vi "Create AO waveforms Parallel.vi"(9 "sampling info":cluster{"Fs":dbl, "#s":dbl}={"Fs"=1000.0, "#s"=1000.0} {"Fs" format="%.2p"}, 10 "reset signal":bool, 11 "Cluster":T1={"AO amp (V)"=[0.001, 2e-08, 0.001, 0.001, 0.001, 2e-08, 0.0, 0.0], "AO DC (V)"=[0.0, 0.0, 0.0, 0.0, 0.0, 0.0, 0.0, 0.0], "AO f (Hz)"=[13.0, 13.0, 13.0, 13.0, 13.0, 13.0, 13.0, 13.0], "AO phi (deg)"=[0.0, 0.0, 0.0, 0.0, 0.0, 0.0, 0.0, 0.0], "REF f (Hz)"=[13.0, 13.0, 13.0, 13.0, 13.0, 13.0, 13.0, 13.0], "function"=[enum."Sine Wave", enum."Sine Wave", enum."Sine Wave", enum."Sine Wave", enum."Sine Wave", enum."Sine Wave", enum."Sine Wave", enum."Sine Wave"], "REF phi (deg)"=[0.0, 0.0, 0.0, 0.0, 0.0, 0.0, 0.0, 0.0]} {"AO DC (V)" format="%#_6p"; "AO amp (V)" format="%#_6p"}) -> (1 "AO Array":waveform(dbl)[](array[waveform]))   [LabVIEW 2013]
uses:
  <vilib>/measure/NI_MABase.lvlib
panel:
  out "Cluster out":T1={"AO amp (V)"=[0.001, 2e-08, 0.001, 0.001, 0.001, 2e-08, 0.0, 0.0], "AO DC (V)"=[0.0, 0.0, 0.0, 0.0, 0.0, 0.0, 0.0, 0.0], "AO f (Hz)"=[13.0, 13.0, 13.0, 13.0, 13.0, 13.0, 13.0, 13.0], "AO phi (deg)"=[0.0, 0.0, 0.0, 0.0, 0.0, 0.0, 0.0, 0.0], "REF f (Hz)"=[13.0, 13.0, 13.0, 13.0, 13.0, 13.0, 13.0, 13.0], "function"=[enum."Sine Wave", enum."Sine Wave", enum."Sine Wave", enum."Sine Wave", enum."Sine Wave", enum."Sine Wave", enum."Sine Wave", enum."Sine Wave"], "REF phi (deg)"=[0.0, 0.0, 0.0, 0.0, 0.0, 0.0, 0.0, 0.0]} {"AO DC (V)" format="%#_6p"; "AO amp (V)" format="%#_6p"}
  out "Waveform Graph":waveform(dbl)[](graph)
  out "phase out":dbl[](array[numeric])
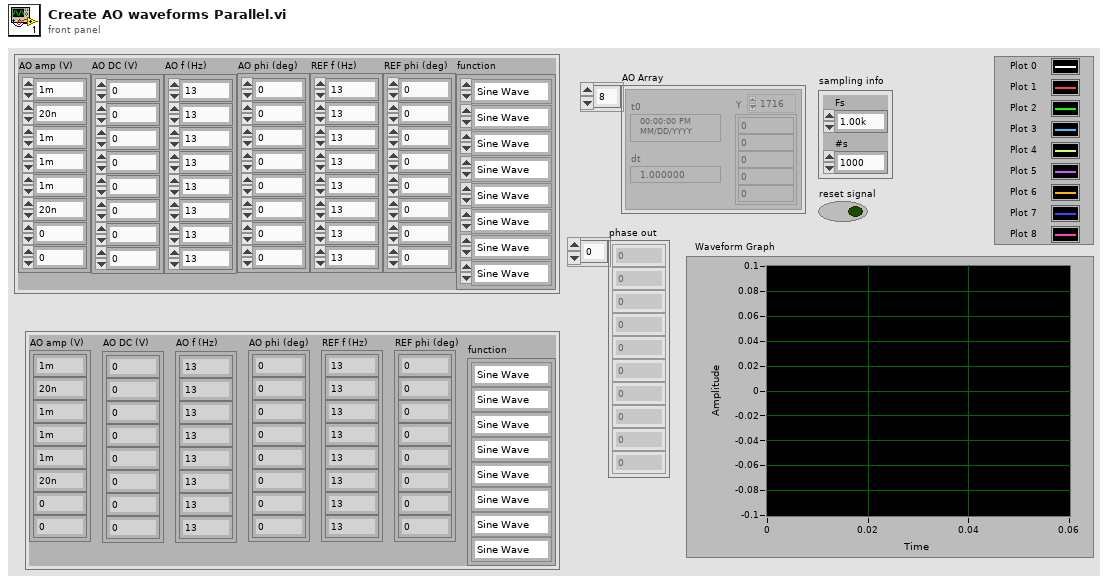
[diagram p1: front panel]
types:
  T1 = cluster{"AO amp (V)":dbl[], "AO DC (V)":dbl[], "AO f (Hz)":dbl[], "AO phi (deg)":dbl[], "REF f (Hz)":dbl[], "function":enum16{"Sine Wave", "Triangle Wave", "Square Wave", "Sawtooth Wave"}[], "REF phi (deg)":dbl[]}
  T2 = enum16{"Sine Wave", "Triangle Wave", "Square Wave", "Sawtooth Wave"}[]
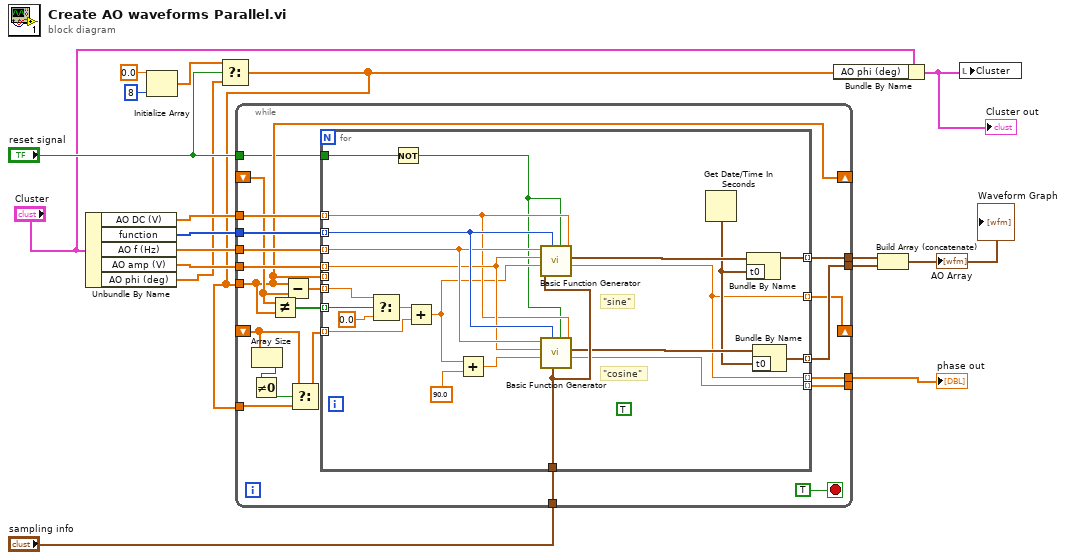
[diagram p0: block diagram]
diagram:
  n1 = Unbundle By Name("Cluster") -> ("AO DC (V)"=w17:dbl[], "function"=w18:T2, "AO f (Hz)"=w13:dbl[], "AO amp (V)"=w14:dbl[], "AO phi (deg)"=w7:dbl[])
  n2 = Initialize Array(0.0 ("element"), 8 ("dimension size")) -> (w9:dbl[])
  n3 = Select(t=w9, s="reset signal", f=w7) -> (s? t:f=w6:dbl[])
  n4 = while {
    tunnel: w18 -> [w39]
    tunnel: w17 -> [w38]
    tunnel: "sampling info" -> [w37]
    tunnel: [w36] -> w4
    tunnel: [w35] -> w15
    tunnel: w14 -> [w34]
    tunnel: w6 -> [w26]
    tunnel: w13 -> [w33]
    tunnel: [w31] -> w12
    tunnel: [w30] -> w1
    shift-right: [w26] -> _
    shift-left: _ -> [w28]
    shift-right: [w25] -> _
    shift-left: _ -> [w20]
    tunnel: w6 -> [w21]
    tunnel: "reset signal" -> [w19]
    stop <- TRUE stop-if-true
    n5 = Array Size(array=w20) -> (size(s)=w23:i32)
    n6 = Not Equal To 0?(x=w23) -> (x != 0?=w22:bool)
    n7 = Not Equal?(x=w28, y=w26) -> (x != y?=w29:bool[])
    n8 = Subtract(x=w26, y=w28) -> (x-y=w27:dbl[])
    n9 = Select(t=w20, s=w22, f=w21) -> (s? t:f=w24:dbl[])
    n10 = for {
      tunnel: w39 -> [w61] mode=indexing
      tunnel: w33 -> [w60] mode=indexing
      tunnel: w34 -> [w59] mode=indexing
      tunnel: w38 -> [w58] mode=indexing
      tunnel: [w55] -> w36 mode=indexing
      tunnel: w37 -> [w57]
      tunnel: [w54] -> w35 mode=indexing
      tunnel: [w49] -> w30 mode=indexing
      tunnel: [w51] -> w31 mode=indexing
      tunnel: w29 -> [w42] mode=indexing
      tunnel: w27 -> [w46] mode=indexing
      tunnel: w26 -> [_] mode=indexing
      tunnel: [w49] -> w25 mode=indexing
      tunnel: w24 -> [w47] mode=indexing
      tunnel: w19 -> [w41]
      (unwired) TRUE
      # "\"cosine\""
      # "\"sine\""
      n11 = Select(t=w46, s=w42, f=0.0) -> (s? t:f=w48:dbl)
      n12 = Not(x=w41) -> (.not. x?=w40:bool)
      n13 = Add(x=w48, y=w47) -> (x+y=w43:dbl)
      n14 = Add(x=w43, y=90.0) -> (x+y=w44:dbl)
      n15 = call <vilib>:"Basic Function Generator.vi"("offset"=w58, "reset signal"=w40, "sampling info"=w57, "signal type"=w61, "phase"=w43, "amplitude"=w59, "frequency"=w60) -> ("phase out"=w49:dbl, "signal out"=w56:waveform(dbl))  [unwired: 2 in, 1 out]
      n16 = call <vilib>:"Basic Function Generator.vi"("offset"=w58, "reset signal"=w40, "sampling info"=w57, "signal type"=w61, "phase"=w44, "amplitude"=w59, "frequency"=w60) -> ("phase out"=w51:dbl, "signal out"=w53:waveform(dbl))  [unwired: 2 in, 1 out]
      n17 = Get Date/Time In Seconds() -> (seconds since 1Jan1904=w52:timestamp)
      n18 = Bundle By Name(cluster=w56, "t0"=w52) -> (w55:waveform(dbl))
      n19 = Bundle By Name(cluster=w53, "t0"=w52) -> (w54:waveform(dbl))
    }
  }
  "phase out" <- w1
  n20 = Bundle By Name(cluster="Cluster", "AO phi (deg)"=w6) -> (w2:T1)
  "Cluster out" <- w2
  n21 = Build Array (concatenate)(w4, w15) -> (→"AO Array" →"Waveform Graph":waveform(dbl)[])
  n22 = local write "Cluster"(w2) -> ()
